vi "Real Wind Monitor.vi"() -> ()   [LabVIEW 2026]
uses:
  Real Wind Sample.ctl
  <vilib>/Instr/_visa.llb/VISA Configure Serial Port (Instr).vi
panel:
  out "ID Gap?":bool
  out "Packet Intervals":u64(graph)
  out "Current Record ID":u64
  out "Whole Packet":string
  out "CSV Log?":bool
  out "VISA Errors":errorcluster
  in  "Choose:":refnum<visa-resource-name>
  out "Direction Parsed":string
  out "Error Logs:":errorcluster
  out "CSV File Path/Row Preview":string
  in  "CSV File Path":path
  in  "Enable Logging?":bool
  out "Wind Speed History":dbl(graph)
  out "Wind Direction History":dbl(graph)
  out "All Valid?":bool
  out "Current Wind Sample:":T1
  out "Speed Parsed":string
  in  "?":bool
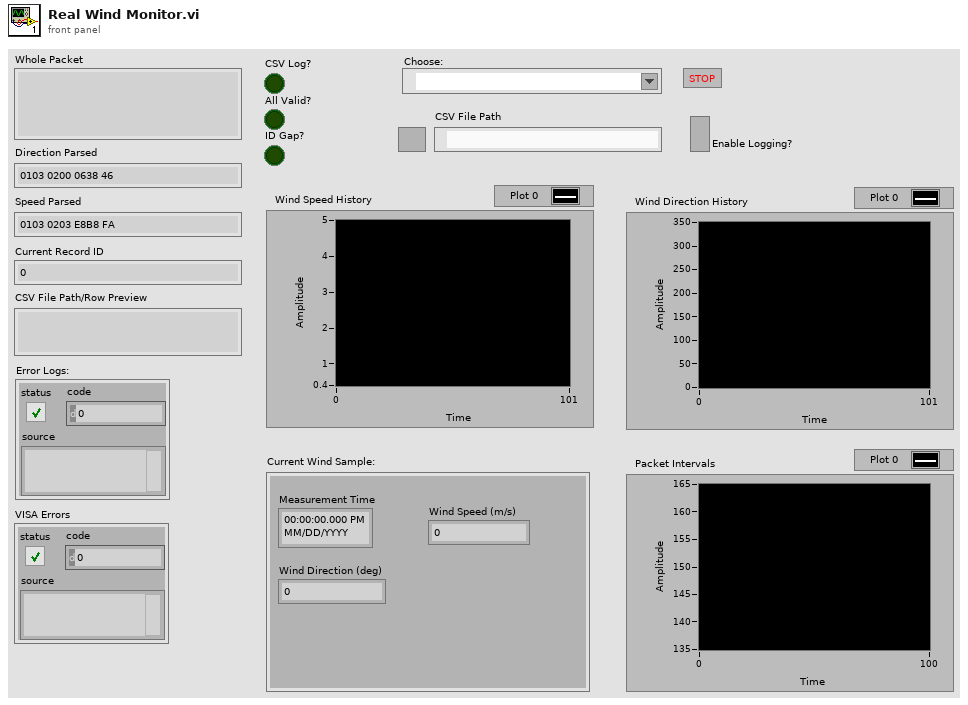
[diagram p1: front panel]
types:
  T1 = typedef "Real Wind Sample.ctl" = cluster{"Measurement Time":timestamp, "Wind Direction (deg)":dbl, "Wind Speed (m/s)":dbl}
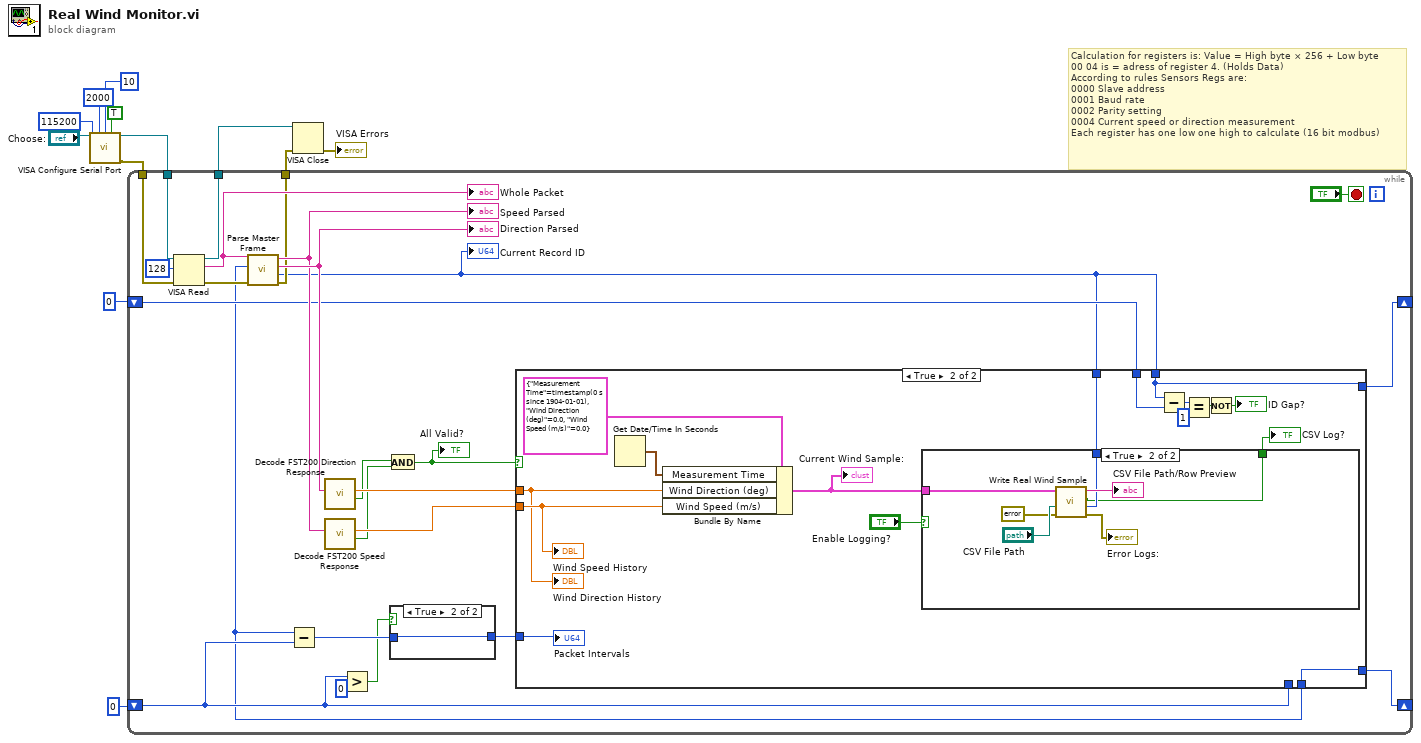
[diagram p0: block diagram]
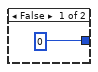
[diagram p2: hidden frame]
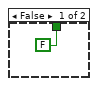
[diagram p4: hidden frame]
diagram:
  # "Calculation for registers is: Value = High byte × 256 + Low byte\n00 04 is = adress of register 4. (Holds Data)\nAccording to rules Sensors Regs are: \n0000\tSlave address\n0001\tBaud rate\n0002\tParity setting\n0004\tCurrent speed or direction measurement\nEach register has one low one high to calculate (16 bit modbus)"
  n1 = call-poly "VISA Configure Serial Port"("VISA resource name"="Choose:", "timeout (10sec)"=u32 2000, "termination char\n(0xA = '\\n' = LF)"=u8 10 ("termination char\n(0xA = '\\n' = LF)"), "Enable Termination\nChar (T)"=TRUE ("Enable Termination\nChar (T)"), "baud rate (9600)"=u32 115200) -> ("VISA resource name out"=w3:refnum<visa-resource-name>, "error out"=w4:errorcluster)  [unwired: 9 in]
  n2 = while {
    shift-right: [w13] -> _
    shift-left: u64 0 -> [w31]
    shift-right: [w16] -> _
    shift-left: u64 0 -> [w26]
    tunnel: w4 -> [w29]
    tunnel: w3 -> [w28]
    tunnel: [w25] -> w2
    tunnel: [w22] -> w1
    stop <- "?" stop-if-true
    n3 = VISA Read(VISA resource name=w28, byte count=u32 128, error in (no error)=w29) -> (VISA resource name out=w25:refnum<visa-resource-name>, read buffer=w23:string, error out=w27:errorcluster)  [unwired: 1 out]
    "Whole Packet" <- w23
    n4 = call "Parse Master Frame.vi"("error in (no error)"=w27, "Raw Master Line"=w23) -> ("error out"=w22:errorcluster, "Record ID"=w19:u64, "direction frame"=w34:string, "speed frame"=w33:string, "TIMESTAMP"=w24:u64)  [unwired: 5 in]
    "Speed Parsed" <- w33
    "Direction Parsed" <- w34
    "Current Record ID" <- w19
    n5 = Subtract(x=w24, y=w31) -> (x-y=w32:u64)
    n6 = call "Decode FST200 Direction Response.vi"("Direction Modbus Response"=w34) -> ("Frame Valid?"=w18:bool, "Wind Direction (deg)"=w36:dbl)  [unwired: 9 in]
    n7 = call "Decode FST200 Speed Response.vi"("Modbus Response"=w33) -> ("Frame Valid?"=w17:bool, "Wind Speed (m/s)"=w21:dbl)  [unwired: 9 in]
    n8 = Greater?(x=w31, y=u64 0 ("x")) -> (0:w14:bool)
    n9 = And(x=w18, y=w17) -> (x .and. y?=w20:bool)
    "All Valid?" <- w20
    n10 = case shown="True" w14 {
      tunnel: w32 -> [_ w39]
      tunnel: [0 w39] -> w15
      frame False {
      }
      frame True {
      }
    }
    n11 = case shown="True" w20 {
      tunnel: w21 -> [_ w56]
      tunnel: w36 -> [_ w53]
      tunnel: w19 -> [_ w52]
      tunnel: [w41 w51] -> w13
      tunnel: w24 -> [_ w51]
      tunnel: w31 -> [w41 _]
      tunnel: w26 -> [w40 w48]
      tunnel: w19 -> [_ w42]
      tunnel: [w40 w42] -> w16
      tunnel: w15 -> [_ w43]
      frame False {
      }
      frame True {
        n12 = Get Date/Time In Seconds() -> (seconds since 1Jan1904=w55:timestamp)
        n13 = Bundle By Name(cluster=T1 {"Measurement Time"=timestamp(0 s since 1904-01-01), "Wind Direction (deg)"=0.0, "Wind Speed (m/s)"=0.0} ("Real Wind Sample"), "Measurement Time"=w55, "Wind Direction (deg)"=w53, "Wind Speed (m/s)"=w56) -> (w46:T1)
        "Current Wind Sample:" <- w46
        n14 = case shown="True" "Enable Logging?" {
          tunnel: w46 -> [_ w65]
          tunnel: w52 -> [_ w60]
          tunnel: [FALSE w59] -> w45
          frame False {
          }
          frame True {
            n15 = call "Write Real Wind Sample.vi"("Record ID"=w60, "error in"=errorcluster {"status"=FALSE, "code"=0, "source"=""}, "CSV File Path"="CSV File Path", "Real Wind Sample"=w65) -> ("error out"=→"Error Logs:":errorcluster, "Csv Commit OKK?"=w59:bool, "CSV Row Preview"=→"CSV File Path/Row Preview":string)  [unwired: 1 in]
          }
        }
        "CSV Log?" <- w45
        n16 = Subtract(x=w42, y=w48) -> (x-y=w50:u64)
        n17 = Equal?(x=w50, y=u64 1) -> (x = y?=w47:bool)
        n18 = Not(x=w47) -> (.not. x?=→"ID Gap?":bool)
        "Wind Direction History" <- w53
        "Wind Speed History" <- w56
        "Packet Intervals" <- w43
      }
    }
  }
  n19 = VISA Close(VISA resource name=w2, error in (no error)=w1) -> (error out=→"VISA Errors":errorcluster)
